vi "Calculate analog channels MUX80.vi"(0 "Channels In":string[](array[string])=["0", "1", "2", "3", "4", "5", "6", "7"]) -> (1 "Channels Out":string[](array[string])=["0", "1", "2", "3", "4", "5", "6", "7"], 2 "Channel Converted?":bool[](array[boolean]))   [LabVIEW 2020]
panel:
  # "The purpose of this vi is to convert an array of string channel names to their corresponding AIN channel number\nfor use with a CB37 and MUX80. The input strings should be of the form Xn-AIN/DAC/FIOn. For example, an input \nof X4-FIO6 would correspond to a CB37 connected to X4 on the MUX80 and a signal connected to FIO6 on the CB37.\nThis would then be translated to the number  94 as it corresponds to AIN94. \n\nSee https://labjack.com/support/datasheets/accessories/mux80 for  more information on this conversion."
  # "Input format: X4-FIO6"
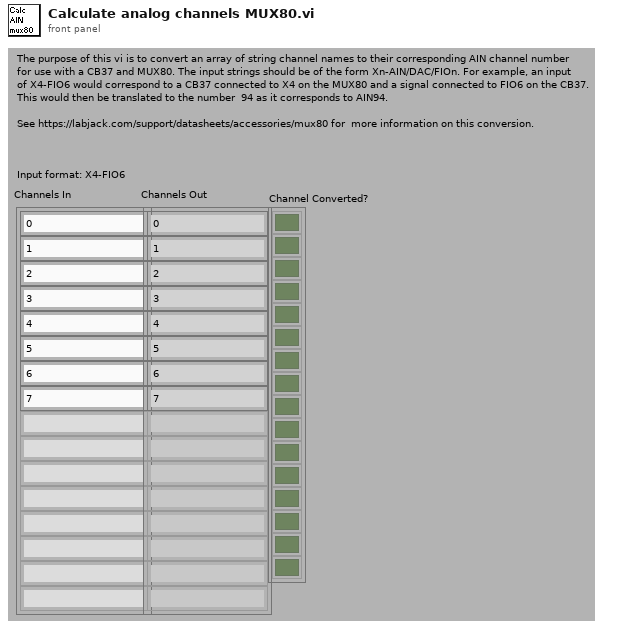
[diagram p1: front panel]
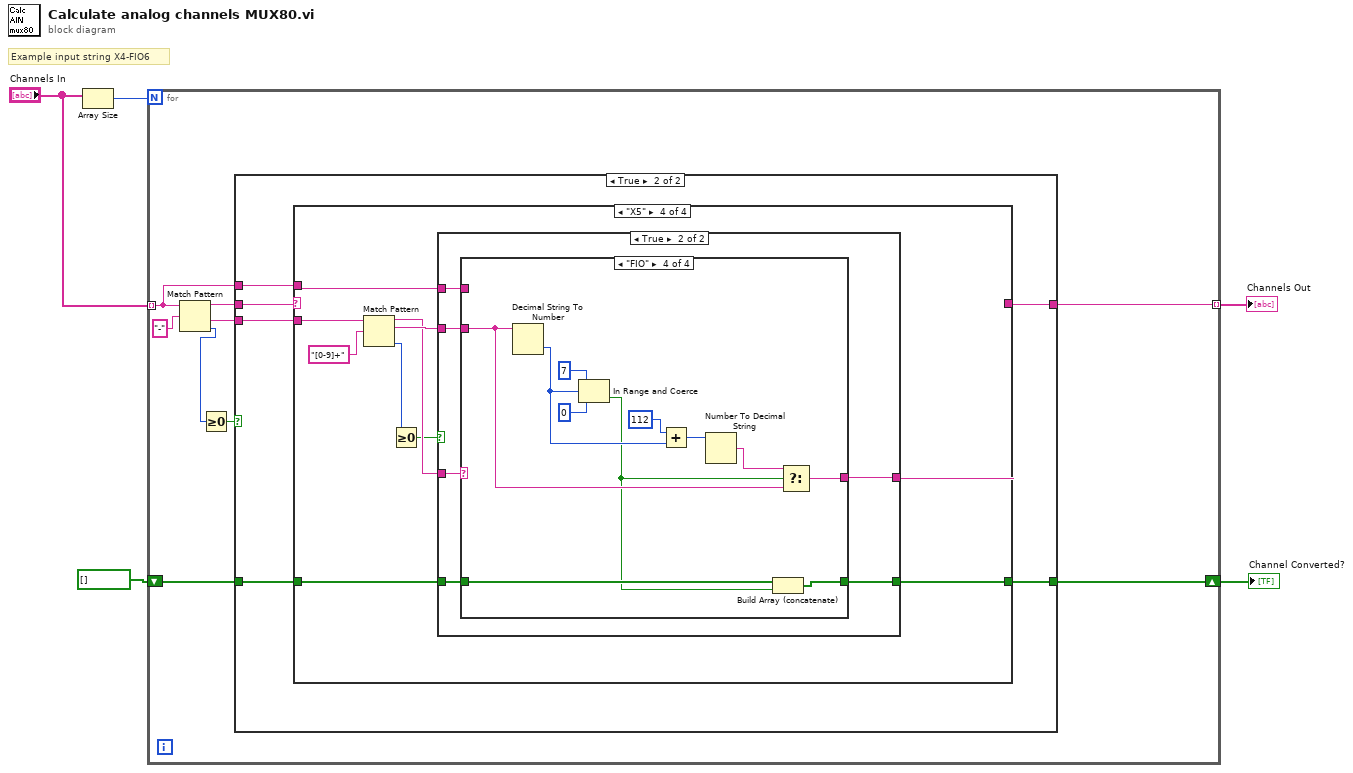
[diagram p0: block diagram]
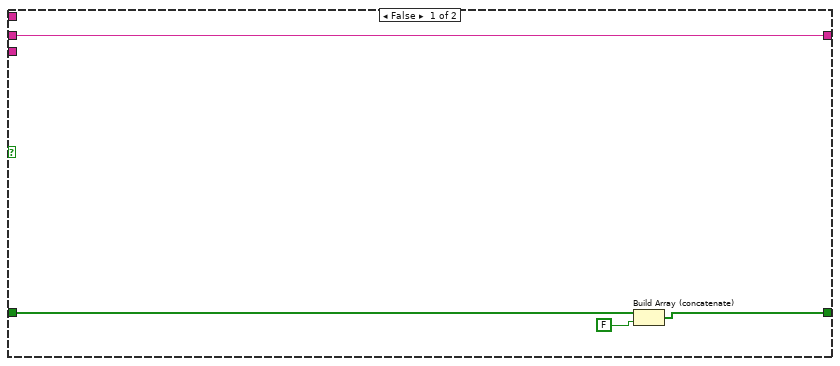
[diagram p2: hidden frame]
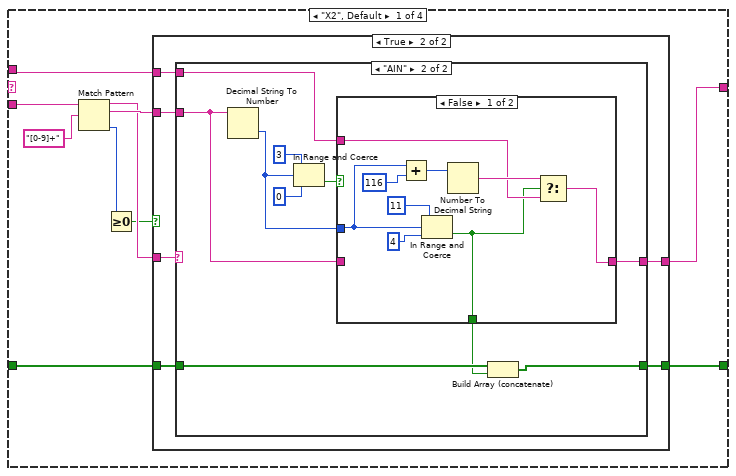
[diagram p3: hidden frame]
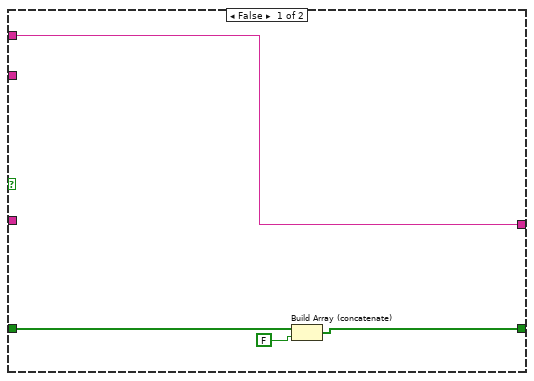
[diagram p4: hidden frame]
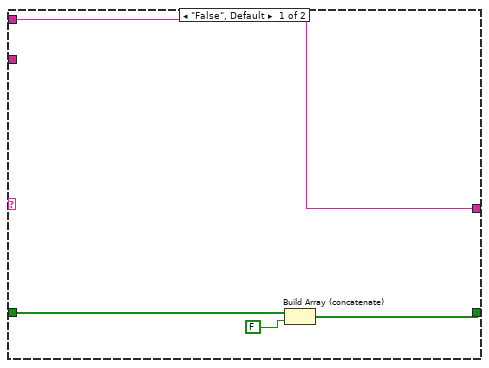
[diagram p5: hidden frame]
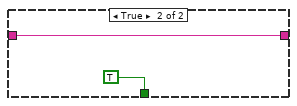
[diagram p6: hidden frame]
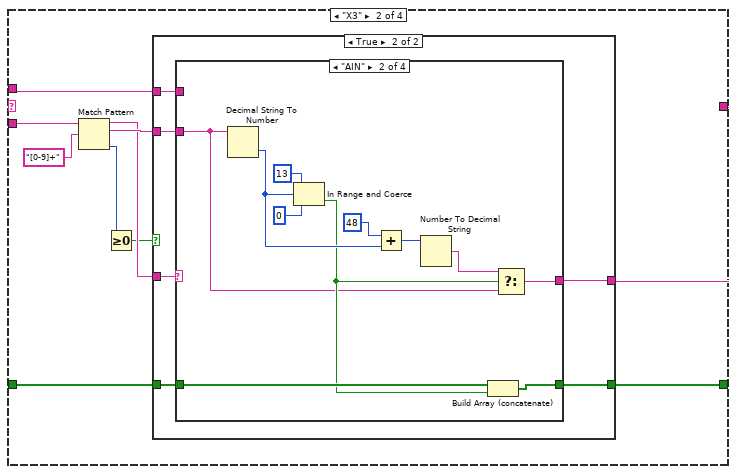
[diagram p7: hidden frame]
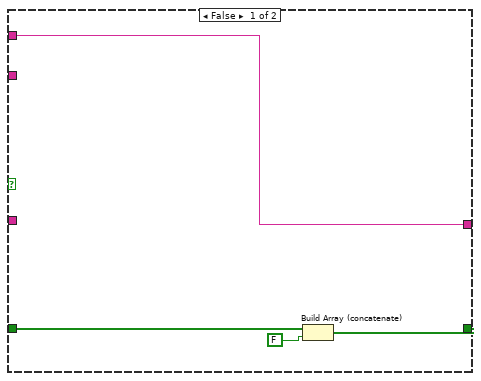
[diagram p8: hidden frame]
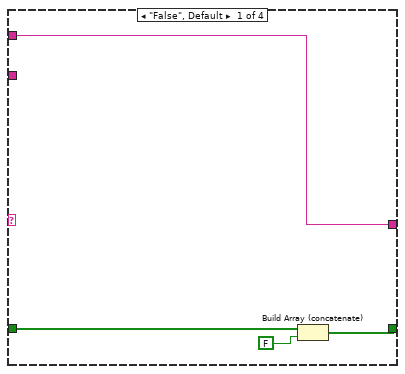
[diagram p9: hidden frame]
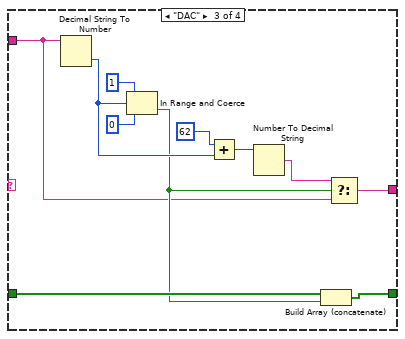
[diagram p10: hidden frame]
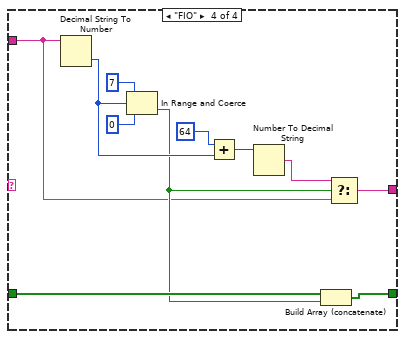
[diagram p11: hidden frame]
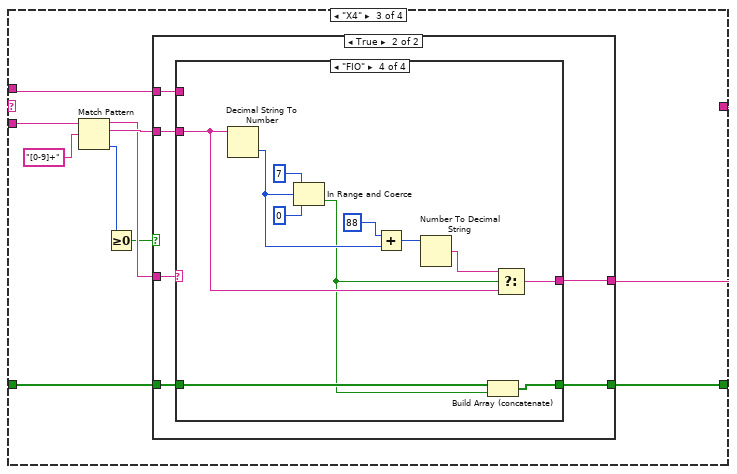
[diagram p12: hidden frame]
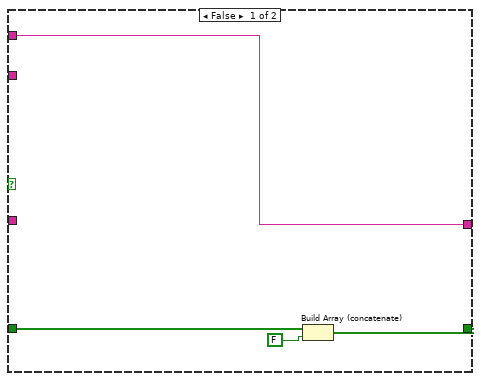
[diagram p13: hidden frame]
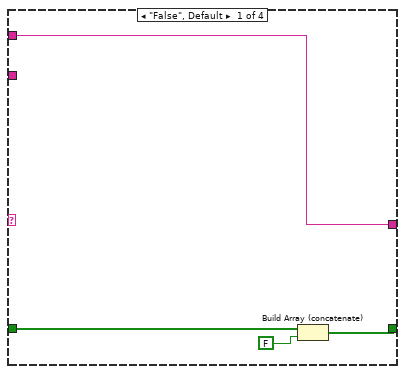
[diagram p14: hidden frame]
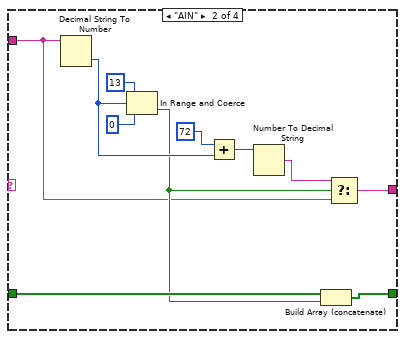
[diagram p15: hidden frame]
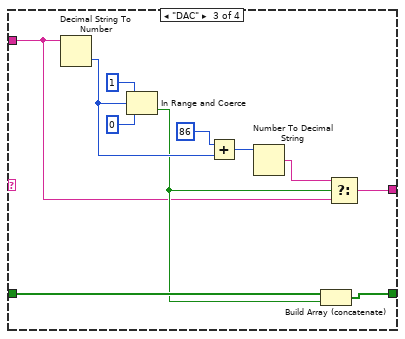
[diagram p16: hidden frame]
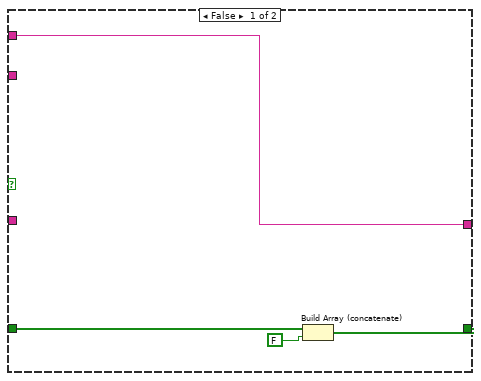
[diagram p17: hidden frame]
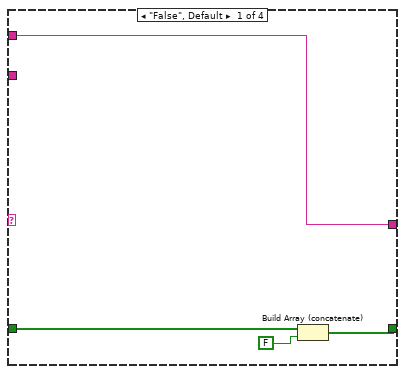
[diagram p18: hidden frame]
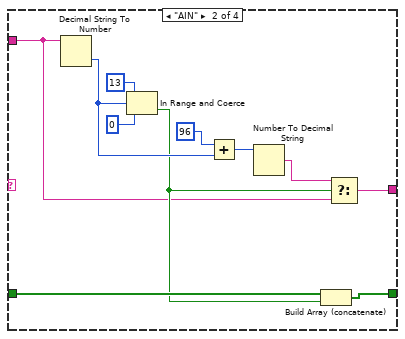
[diagram p19: hidden frame]
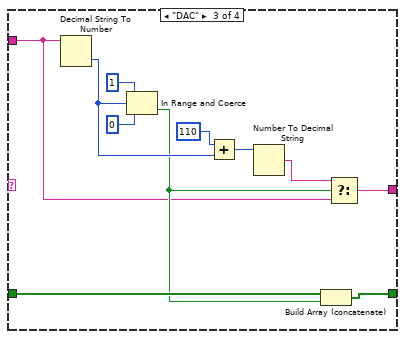
[diagram p20: hidden frame]
diagram:
  # "Example input string X4-FIO6"
  n1 = Array Size(array="Channels In") -> (size(s)=w5:i32)
  n2 = for {
    N: w5 -> [_]
    tunnel: "Channels In" -> [w9] mode=indexing
    shift-right: [w7] -> w2
    shift-left: bool[] [] -> [w8]
    tunnel: [w6] -> w1 mode=indexing
    n3 = Match Pattern(string=w9, regular expression="-") -> (before substring=w11:string, after substring=w10:string, offset past match=w12:i32)  [unwired: 1 in, 1 out]
    n4 = Greater Or Equal To 0?(x=w12) -> (x >= 0?=w13:bool)
    n5 = case shown="True" w13 {
      tunnel: w11 -> [w18 w24]
      tunnel: [w18 w22] -> w6
      tunnel: w10 -> [_ w23]
      tunnel: w9 -> [_ w21]
      tunnel: w8 -> [w17 w20]
      tunnel: [w15 w19] -> w7
      frame False {
        n6 = Build Array (concatenate)(w17, FALSE) -> (w15:bool[])
      }
      frame True {
        n7 = case shown="\"X5\"" w24 {
          tunnel: w23 -> [w33 w78 w135 w192]
          tunnel: [w34 w79 w136 w193] -> w22
          tunnel: w21 -> [w29 w74 w131 w188]
          tunnel: w20 -> [w26 w71 w128 w185]
          tunnel: [w25 w70 w127 w184] -> w19
          frame "X2", Default {
            n8 = Match Pattern(string=w33, regular expression="[0-9]+") -> (before substring=w30:string, match substring=w31:string, offset past match=w28:i32)  [unwired: 1 in, 1 out]
            n9 = Greater Or Equal To 0?(x=w28) -> (x >= 0?=w27:bool)
            n10 = case shown="True" w27 {
              tunnel: [w38 w44] -> w34
              tunnel: w31 -> [_ w43]
              tunnel: w30 -> [_ w42]
              tunnel: w29 -> [w38 w41]
              tunnel: w26 -> [w37 w40]
              tunnel: [w35 w39] -> w25
              frame False {
                n11 = Build Array (concatenate)(w37, FALSE) -> (w35:bool[])
              }
              frame True {
                n12 = case shown="\"AIN\"" w42 {
                  tunnel: [w48 w54] -> w44
                  tunnel: w43 -> [_ w53]
                  tunnel: w41 -> [w48 w49]
                  tunnel: w40 -> [w47 w52]
                  tunnel: [w46 w50] -> w39
                  frame "False", Default {
                    n13 = Build Array (concatenate)(w47, FALSE) -> (w46:bool[])
                  }
                  frame "AIN" {
                    n14 = Decimal String To Number(string=w53) -> (number=w55:i32)  [unwired: 2 in, 1 out]
                    n15 = In Range and Coerce(upper limit=3, x=w55, lower limit=0) -> (In Range?=w56:bool)  [unwired: 1 out]
                    n16 = case shown="False" w56 {
                      tunnel: w55 -> [w64 _]
                      tunnel: [w59 w69] -> w54
                      tunnel: w53 -> [_ w69]
                      tunnel: [w60 TRUE] -> w51
                      tunnel: w49 -> [w61 _]
                      frame False {
                        n17 = Add(x=w64, y=116) -> (x+y=w63:i32)
                        n18 = In Range and Coerce(upper limit=11, x=w64, lower limit=4) -> (In Range?=w60:bool)  [unwired: 1 out]
                        n19 = Number To Decimal String(number=w63) -> (decimal integer string=w62:string)  [unwired: 1 in]
                        n20 = Select(t=w62, s=w60, f=w61) -> (s? t:f=w59:string)
                      }
                      frame True {
                      }
                    }
                    n21 = Build Array (concatenate)(w52, w51) -> (w50:bool[])
                  }
                }
              }
            }
          }
          frame "X3" {
            n22 = Match Pattern(string=w78, regular expression="[0-9]+") -> (before substring=w75:string, match substring=w76:string, offset past match=w73:i32)  [unwired: 1 in, 1 out]
            n23 = Greater Or Equal To 0?(x=w73) -> (x >= 0?=w72:bool)
            n24 = case shown="True" w72 {
              tunnel: [w83 w89] -> w79
              tunnel: w76 -> [_ w88]
              tunnel: w75 -> [_ w87]
              tunnel: w74 -> [w83 w86]
              tunnel: w71 -> [w82 w85]
              tunnel: [w80 w84] -> w70
              frame False {
                n25 = Build Array (concatenate)(w82, FALSE) -> (w80:bool[])
              }
              frame True {
                n26 = case shown="\"AIN\"" w87 {
                  tunnel: [w93 w94 w105 w116] -> w89
                  tunnel: w88 -> [_ w95 w106 w117]
                  tunnel: w86 -> [w93 _ _ _]
                  tunnel: w85 -> [w92 w101 w112 w123]
                  tunnel: [w91 w100 w111 w122] -> w84
                  frame "False", Default {
                    n27 = Build Array (concatenate)(w92, FALSE) -> (w91:bool[])
                  }
                  frame "AIN" {
                    n28 = Decimal String To Number(string=w95) -> (number=w102:i32)  [unwired: 2 in, 1 out]
                    n29 = In Range and Coerce(upper limit=13, x=w102, lower limit=0) -> (In Range?=w96:bool)  [unwired: 1 out]
                    n30 = Add(x=48, y=w102) -> (x+y=w98:i32)
                    n31 = Number To Decimal String(number=w98) -> (decimal integer string=w97:string)  [unwired: 1 in]
                    n32 = Build Array (concatenate)(w101, w96) -> (w100:bool[])
                    n33 = Select(t=w97, s=w96, f=w95) -> (s? t:f=w94:string)
                  }
                  frame "DAC" {
                    n34 = Decimal String To Number(string=w106) -> (number=w113:i32)  [unwired: 2 in, 1 out]
                    n35 = In Range and Coerce(upper limit=1, x=w113, lower limit=0) -> (In Range?=w107:bool)  [unwired: 1 out]
                    n36 = Add(x=62, y=w113) -> (x+y=w109:i32)
                    n37 = Number To Decimal String(number=w109) -> (decimal integer string=w108:string)  [unwired: 1 in]
                    n38 = Build Array (concatenate)(w112, w107) -> (w111:bool[])
                    n39 = Select(t=w108, s=w107, f=w106) -> (s? t:f=w105:string)
                  }
                  frame "FIO" {
                    n40 = Decimal String To Number(string=w117) -> (number=w124:i32)  [unwired: 2 in, 1 out]
                    n41 = In Range and Coerce(upper limit=7, x=w124, lower limit=0) -> (In Range?=w118:bool)  [unwired: 1 out]
                    n42 = Add(x=64, y=w124) -> (x+y=w120:i32)
                    n43 = Number To Decimal String(number=w120) -> (decimal integer string=w119:string)  [unwired: 1 in]
                    n44 = Build Array (concatenate)(w123, w118) -> (w122:bool[])
                    n45 = Select(t=w119, s=w118, f=w117) -> (s? t:f=w116:string)
                  }
                }
              }
            }
          }
          frame "X4" {
            n46 = Match Pattern(string=w135, regular expression="[0-9]+") -> (before substring=w132:string, match substring=w133:string, offset past match=w130:i32)  [unwired: 1 in, 1 out]
            n47 = Greater Or Equal To 0?(x=w130) -> (x >= 0?=w129:bool)
            n48 = case shown="True" w129 {
              tunnel: [w140 w146] -> w136
              tunnel: w133 -> [_ w145]
              tunnel: w132 -> [_ w144]
              tunnel: w131 -> [w140 w143]
              tunnel: w128 -> [w139 w142]
              tunnel: [w137 w141] -> w127
              frame False {
                n49 = Build Array (concatenate)(w139, FALSE) -> (w137:bool[])
              }
              frame True {
                n50 = case shown="\"FIO\"" w144 {
                  tunnel: [w150 w151 w162 w176] -> w146
                  tunnel: w145 -> [_ w152 w163 w174]
                  tunnel: w143 -> [w150 _ _ _]
                  tunnel: w142 -> [w149 w158 w169 w181]
                  tunnel: [w148 w157 w168 w180] -> w141
                  frame "False", Default {
                    n51 = Build Array (concatenate)(w149, FALSE) -> (w148:bool[])
                  }
                  frame "AIN" {
                    n52 = Decimal String To Number(string=w152) -> (number=w159:i32)  [unwired: 2 in, 1 out]
                    n53 = In Range and Coerce(upper limit=13, x=w159, lower limit=0) -> (In Range?=w153:bool)  [unwired: 1 out]
                    n54 = Add(x=72, y=w159) -> (x+y=w155:i32)
                    n55 = Number To Decimal String(number=w155) -> (decimal integer string=w154:string)  [unwired: 1 in]
                    n56 = Build Array (concatenate)(w158, w153) -> (w157:bool[])
                    n57 = Select(t=w154, s=w153, f=w152) -> (s? t:f=w151:string)
                  }
                  frame "DAC" {
                    n58 = Decimal String To Number(string=w163) -> (number=w170:i32)  [unwired: 2 in, 1 out]
                    n59 = In Range and Coerce(upper limit=1, x=w170, lower limit=0) -> (In Range?=w164:bool)  [unwired: 1 out]
                    n60 = Add(x=86, y=w170) -> (x+y=w166:i32)
                    n61 = Number To Decimal String(number=w166) -> (decimal integer string=w165:string)  [unwired: 1 in]
                    n62 = Build Array (concatenate)(w169, w164) -> (w168:bool[])
                    n63 = Select(t=w165, s=w164, f=w163) -> (s? t:f=w162:string)
                  }
                  frame "FIO" {
                    n64 = Decimal String To Number(string=w174) -> (number=w177:i32)  [unwired: 2 in, 1 out]
                    n65 = In Range and Coerce(upper limit=7, x=w177, lower limit=0) -> (In Range?=w173:bool)  [unwired: 1 out]
                    n66 = Add(x=88, y=w177) -> (x+y=w178:i32)
                    n67 = Number To Decimal String(number=w178) -> (decimal integer string=w175:string)  [unwired: 1 in]
                    n68 = Build Array (concatenate)(w181, w173) -> (w180:bool[])
                    n69 = Select(t=w175, s=w173, f=w174) -> (s? t:f=w176:string)
                  }
                }
              }
            }
          }
          frame "X5" {
            n70 = Match Pattern(string=w192, regular expression="[0-9]+") -> (before substring=w189:string, match substring=w190:string, offset past match=w187:i32)  [unwired: 1 in, 1 out]
            n71 = Greater Or Equal To 0?(x=w187) -> (x >= 0?=w186:bool)
            n72 = case shown="True" w186 {
              tunnel: [w197 w203] -> w193
              tunnel: w190 -> [_ w202]
              tunnel: w189 -> [_ w201]
              tunnel: w188 -> [w197 w200]
              tunnel: w185 -> [w196 w199]
              tunnel: [w194 w198] -> w184
              frame False {
                n73 = Build Array (concatenate)(w196, FALSE) -> (w194:bool[])
              }
              frame True {
                n74 = case shown="\"FIO\"" w201 {
                  tunnel: [w207 w208 w219 w231] -> w203
                  tunnel: w202 -> [_ w209 w220 w232]
                  tunnel: w200 -> [w207 _ _ _]
                  tunnel: w199 -> [w206 w215 w226 w237]
                  tunnel: [w205 w214 w225 w236] -> w198
                  frame "False", Default {
                    n75 = Build Array (concatenate)(w206, FALSE) -> (w205:bool[])
                  }
                  frame "AIN" {
                    n76 = Decimal String To Number(string=w209) -> (number=w216:i32)  [unwired: 2 in, 1 out]
                    n77 = In Range and Coerce(upper limit=13, x=w216, lower limit=0) -> (In Range?=w210:bool)  [unwired: 1 out]
                    n78 = Add(x=96, y=w216) -> (x+y=w212:i32)
                    n79 = Number To Decimal String(number=w212) -> (decimal integer string=w211:string)  [unwired: 1 in]
                    n80 = Build Array (concatenate)(w215, w210) -> (w214:bool[])
                    n81 = Select(t=w211, s=w210, f=w209) -> (s? t:f=w208:string)
                  }
                  frame "DAC" {
                    n82 = Decimal String To Number(string=w220) -> (number=w227:i32)  [unwired: 2 in, 1 out]
                    n83 = In Range and Coerce(upper limit=1, x=w227, lower limit=0) -> (In Range?=w221:bool)  [unwired: 1 out]
                    n84 = Add(x=110, y=w227) -> (x+y=w223:i32)
                    n85 = Number To Decimal String(number=w223) -> (decimal integer string=w222:string)  [unwired: 1 in]
                    n86 = Build Array (concatenate)(w226, w221) -> (w225:bool[])
                    n87 = Select(t=w222, s=w221, f=w220) -> (s? t:f=w219:string)
                  }
                  frame "FIO" {
                    n88 = Decimal String To Number(string=w232) -> (number=w238:i32)  [unwired: 2 in, 1 out]
                    n89 = In Range and Coerce(upper limit=7, x=w238, lower limit=0) -> (In Range?=w230:bool)  [unwired: 1 out]
                    n90 = Add(x=112, y=w238) -> (x+y=w234:i32)
                    n91 = Number To Decimal String(number=w234) -> (decimal integer string=w233:string)  [unwired: 1 in]
                    n92 = Build Array (concatenate)(w237, w230) -> (w236:bool[])
                    n93 = Select(t=w233, s=w230, f=w232) -> (s? t:f=w231:string)
                  }
                }
              }
            }
          }
        }
      }
    }
  }
  "Channel Converted?" <- w2
  "Channels Out" <- w1
